vi "Power Accuracy Limit Key Array.vi"(4 "Conversion":enum16{"Cluster - HTML", "HTML - Cluster"}(ring), 6 "Limits Key Array In":T2, 7 "Limits Cluster In":T1={"Tolerance"=0.35}) -> (1 "Limits Cluster Out":T1={"Tolerance"=0.35}, 2 "Limits HTML Out":string)   [LabVIEW 2011]
uses:
  Addons/internet/utils/keyedarr.llb/Keyed Array.ctl
  TypeDefs/Power Accuracy Limit Parameters.ctl
  Addons/internet/utils/strutil.llb/Case Matching.ctl
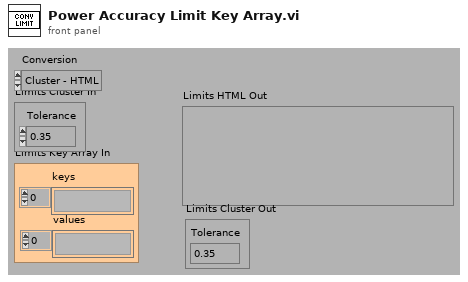
[diagram p1: front panel]
types:
  T1 = typedef "Power Accuracy Limit Parameters.ctl" = cluster{"Tolerance":dbl}
  T2 = typedef "Keyed Array.ctl" = cluster{"keys":string[], "values":string[]}
  T3 = typedef "Case Matching.ctl" = enum16{"a != A", "a == A", "system"}
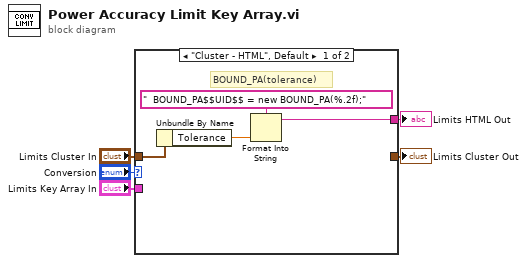
[diagram p0: block diagram]
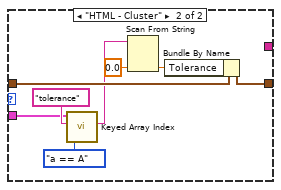
[diagram p2: hidden frame]
diagram:
  n1 = case shown="\"Cluster - HTML\", Default" "Conversion" {
    tunnel: "Limits Key Array In" -> [_ w12]
    tunnel: "Limits Cluster In" -> [w9 w17]
    tunnel: [w6 _] -> w3
    tunnel: [_ w16] -> w2
    frame "Cluster - HTML", Default {
      # "BOUND_PA(tolerance)"
      n2 = Unbundle By Name(w9) -> ("Tolerance"=w7:dbl)
      n3 = Format Into String(format string="  BOUND_PA$$UID$$ = new BOUND_PA(%.2f);", w7) -> (resulting string=w6:string)  [unwired: 2 in, 1 out]
    }
    frame "HTML - Cluster" {
      n4 = call "Keyed Array Index.vi"("case matching (sensitive)"=Case_Matching."a == A", "key"="tolerance", "array in"=w12) -> ("value"=w14:string)  [unwired: 1 in, 3 out]
      n5 = Scan From String(input string=w14, default 1=0.0 ("Display.Power Scale.yRange_min")) -> (output 1=w11:dbl)  [unwired: 3 in, 3 out]
      n6 = Bundle By Name(cluster=w17, "Tolerance"=w11) -> (w16:T1)
    }
  }
  "Limits HTML Out" <- w3
  "Limits Cluster Out" <- w2
